vi "Change Mode Request.vi"(8 "error in (no error)":errorcluster, 9 "Transition time (s)":dbl=1.0 caption="Time Target (s)", 10 "Velocities Norm":dbl[](array[numeric]), 11 "metrics":T1) -> (0 "error out":errorcluster, 2 "Requested?":bool caption="Time has Elapsed", 3 "Robotiq Mode":T2)   [LabVIEW 2011]
uses:
  controls/Robotiq Mode.ctl
  <vilib>/functionblocks/Bistables/RS Bistable/RS Bistable.vi
  <vilib>/functionblocks/FB Core/FB Core.xnode
  <vilib>/functionblocks/NI_FunctionBlock Libraries.lvlib
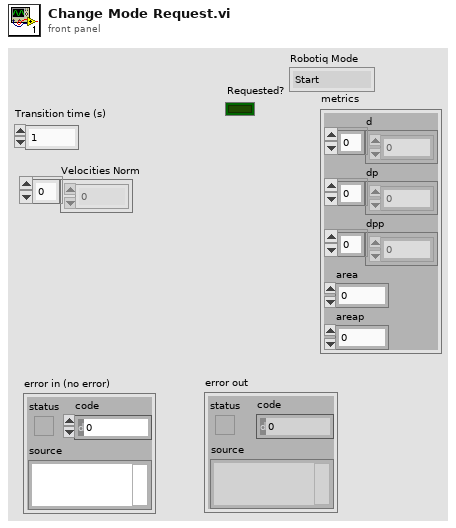
[diagram p1: front panel]
types:
  T1 = cluster{"d":dbl[], "dp":dbl[], "dpp":dbl[], "area":dbl, "areap":dbl}
  T2 = typedef "Robotiq Mode.ctl" = enum16{"Start", "Basic", "Scissor", "Ring", "Pinch"}
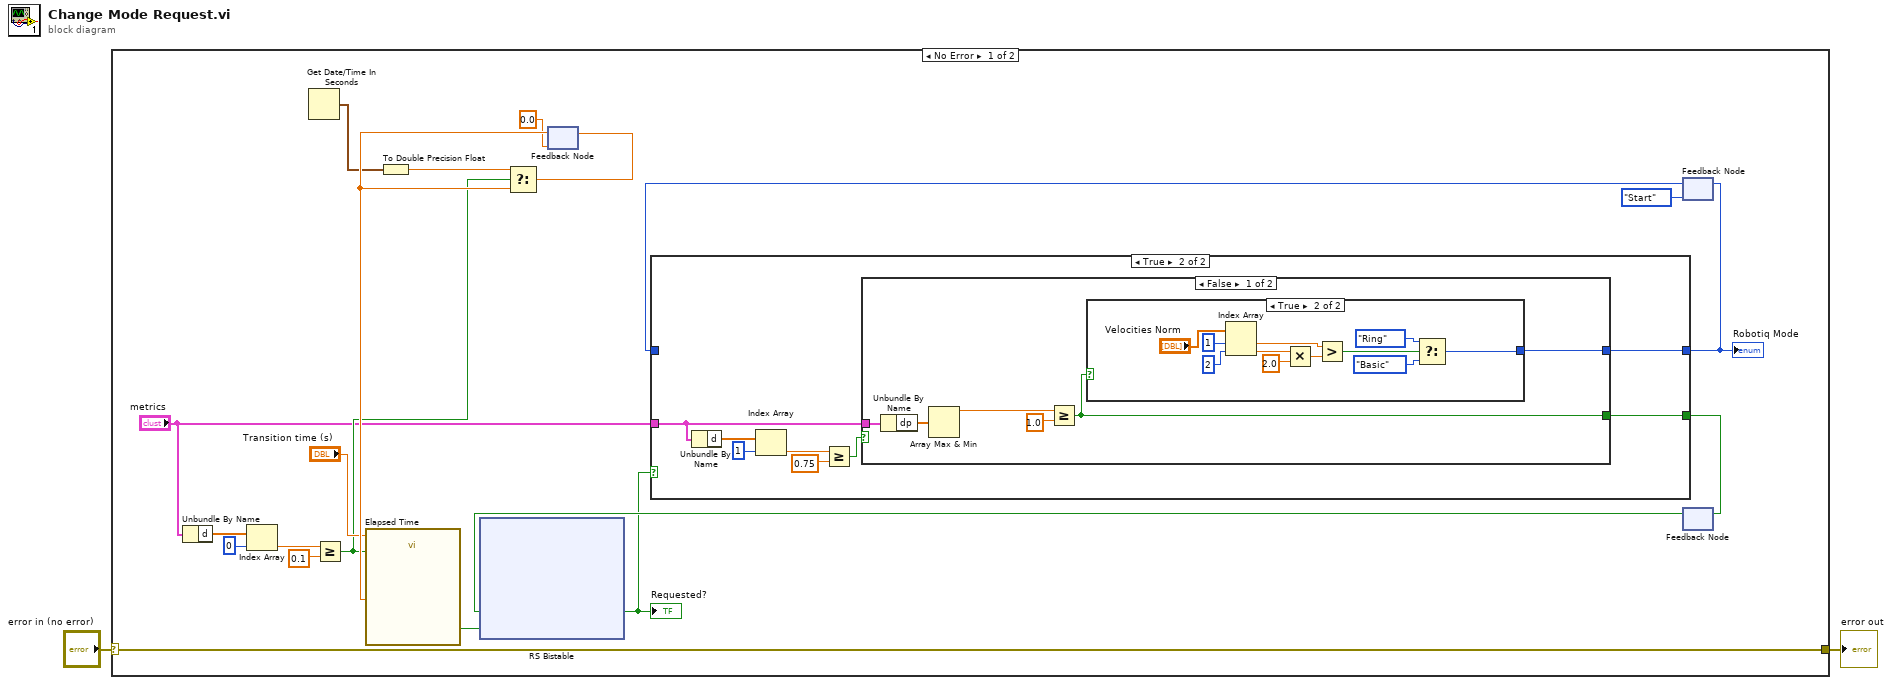
[diagram p0: block diagram]
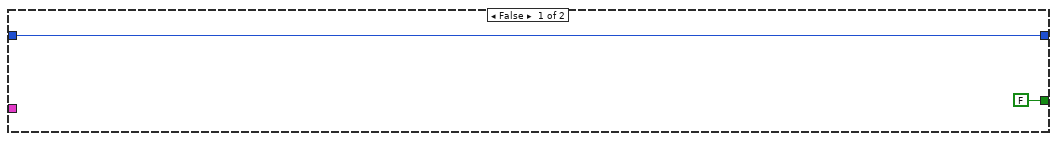
[diagram p2: hidden frame]
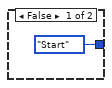
[diagram p3: hidden frame]
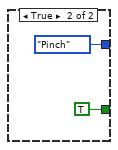
[diagram p4: hidden frame]
diagram:
  n1 = case shown="No Error" "error in (no error)" {
    selector: "error in (no error)" -> [w12 w95]
    tunnel: [w12 w95] -> w1
    frame No Error {
      n2 = Unbundle By Name("metrics") -> ("d"=w14:dbl[])
      n3 = Index Array(array=w14, index=0) -> (element=w13:dbl)
      n4 = Get Date/Time In Seconds() -> (seconds since 1Jan1904=w17:timestamp)
      n5 = Greater Or Equal?(x=w13, y=0.1) -> (x >= y?=w16:bool)
      n6 = To Double Precision Float(number=w17) -> (double precision float=w15:dbl)
      n7 = feedback #1(0.0) -> (w21:dbl)
      n8 = call "Elapsed Time"("Time Target (s)"="Transition time (s)", "Reset"=w16, "Set Start Time (s)"=w21) -> ("Time has Elapsed"=w10:bool)  [unwired: 9 in, 7 out]
      n9 = Select(t=w15, s=w16, f=w21) -> (s? t:f=w22:dbl)
      n10 = feedback-in #1(w22) -> ()
      n11 = feedback #2(Robotiq_Mode."Start" ("Robotiq Mode")) -> (w8:T2)
      n12 = feedback #3() -> (w6:bool)  [unwired: 1 in]
      n13 = xnode "RS Bistable"("reset"=w6, "set"=w10) -> ("output"=w4:bool)  [unwired: 1 in, 1 out]
      "Requested?" <- w4
      n14 = case shown="True" w4 {
        tunnel: "metrics" -> [_ w70]
        tunnel: [w66 w71] -> w9
        tunnel: w8 -> [w66 _]
        tunnel: [FALSE w69] -> w7
        frame False {
        }
        frame True {
          n15 = Unbundle By Name(w70) -> ("d"=w67:dbl[])
          n16 = Index Array(array=w67, index=1) -> (element=w72:dbl)
          n17 = Greater Or Equal?(x=w72, y=0.75) -> (x >= y?=w68:bool)
          n18 = case shown="False" w68 {
            tunnel: [w77 Robotiq_Mode."Pinch" ("Robotiq Mode")] -> w71
            tunnel: w70 -> [w76 _]
            tunnel: [w75 TRUE] -> w69
            frame False {
              n19 = Unbundle By Name(w76) -> ("dp"=w78:dbl[])
              n20 = Array Max & Min(array=w78) -> (max value=w80:dbl)  [unwired: 3 out]
              n21 = Greater Or Equal?(x=w80, y=1.0) -> (x >= y?=w75:bool)
              n22 = case shown="True" w75 {
                tunnel: [Robotiq_Mode."Start" ("Robotiq Mode") w89] -> w77
                frame False {
                }
                frame True {
                  n23 = Index Array(array="Velocities Norm", index #1=1 ("index"), index #2=2 ("index")) -> (element #1=w83:dbl, element #2=w86:dbl)
                  n24 = Multiply(x=w86, y=2.0) -> (x*y=w84:dbl)
                  n25 = Greater?(x=w83, y=w84) -> (0:w82:bool)
                  n26 = Select(t=Robotiq_Mode."Ring" ("Robotiq Mode"), s=w82, f=Robotiq_Mode."Basic" ("Robotiq Mode")) -> (s? t:f=w89:T2)
                }
              }
            }
            frame True {
            }
          }
        }
      }
      "Robotiq Mode" <- w9
      n27 = feedback-in #2(w9) -> ()
      n28 = feedback-in #3(w7) -> ()
    }
    frame Error {
    }
  }
  "error out" <- w1
